vi "Escribir_Fichero_Registro.vi"(0 "refnum FILE":refnum<file>, 1 "ASIC QR CODE":string, 2 "HORA COMIENZO":timestamp, 3 "Coordenada X":string, 4 "Coordenada Y":string, 5 "OPERADOR":string, 6 "Resultado test":bool, 7 "error in (no error)":errorcluster) -> (20 "refnum out":refnum<file>, 27 "error out":errorcluster)   [LabVIEW 2019]
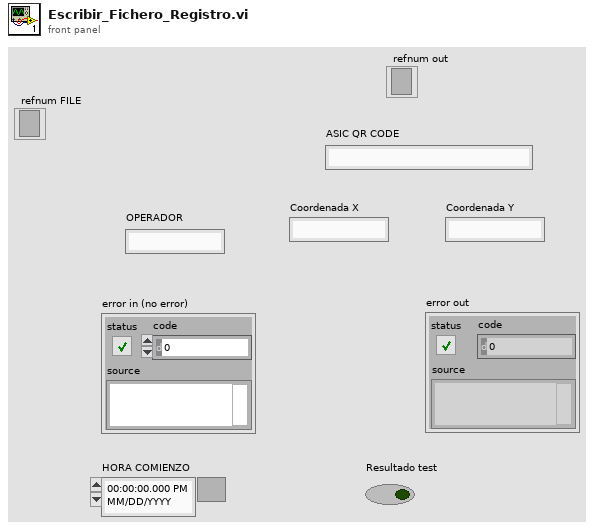
[diagram p1: front panel]
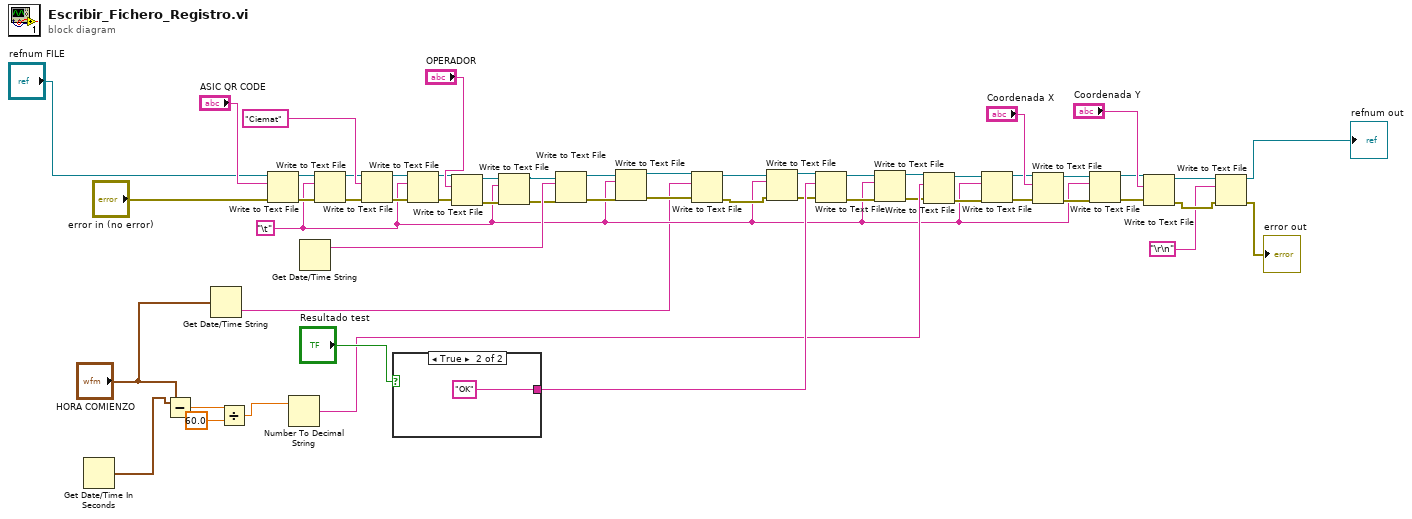
[diagram p0: block diagram]
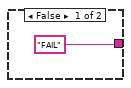
[diagram p2: hidden frame]
diagram:
  w5 = "\t"
  n1 = Get Date/Time In Seconds() -> (seconds since 1Jan1904=w48:timestamp)
  n2 = Subtract(x=w48, y="HORA COMIENZO") -> (x-y=w47:dbl)
  n3 = Get Date/Time String(seconds (now)="HORA COMIENZO") -> (time string=w1:string)  [unwired: 2 in, 1 out]
  n4 = Divide(x=w47, y=60.0) -> (x/y=w45:dbl)
  n5 = Write to Text File(file (use dialog)="refnum FILE", text="ASIC QR CODE", error in="error in (no error)") -> (refnum out=w35:refnum<file>, error out=w34:errorcluster)  [unwired: 1 in, 1 out]
  n6 = Number To Decimal String(number=w45) -> (decimal integer string=w44:string)  [unwired: 1 in]
  n7 = Get Date/Time String() -> (date string=w51:string)  [unwired: 3 in, 1 out]
  n8 = Write to Text File(file (use dialog)=w35, text=w5, error in=w34) -> (refnum out=w33:refnum<file>, error out=w32:errorcluster)  [unwired: 1 in, 1 out]
  n9 = Write to Text File(file (use dialog)=w33, text="Ciemat", error in=w32) -> (refnum out=w31:refnum<file>, error out=w30:errorcluster)  [unwired: 1 in, 1 out]
  n10 = case shown="True" "Resultado test" {
    tunnel: ["FAIL" "OK"] -> w49
    frame False {
    }
    frame True {
    }
  }
  n11 = Write to Text File(file (use dialog)=w31, text=w5, error in=w30) -> (refnum out=w29:refnum<file>, error out=w28:errorcluster)  [unwired: 1 in, 1 out]
  n12 = Write to Text File(file (use dialog)=w29, text="OPERADOR", error in=w28) -> (refnum out=w27:refnum<file>, error out=w26:errorcluster)  [unwired: 1 in, 1 out]
  n13 = Write to Text File(file (use dialog)=w27, text=w5, error in=w26) -> (refnum out=w25:refnum<file>, error out=w24:errorcluster)  [unwired: 1 in, 1 out]
  n14 = Write to Text File(file (use dialog)=w25, text=w51, error in=w24) -> (refnum out=w23:refnum<file>, error out=w22:errorcluster)  [unwired: 1 in, 1 out]
  n15 = Write to Text File(file (use dialog)=w23, text=w5, error in=w22) -> (refnum out=w21:refnum<file>, error out=w20:errorcluster)  [unwired: 1 in, 1 out]
  n16 = Write to Text File(file (use dialog)=w21, text=w1, error in=w20) -> (refnum out=w19:refnum<file>, error out=w18:errorcluster)  [unwired: 1 in, 1 out]
  n17 = Write to Text File(file (use dialog)=w19, text=w5, error in=w18) -> (refnum out=w17:refnum<file>, error out=w16:errorcluster)  [unwired: 1 in, 1 out]
  n18 = Write to Text File(file (use dialog)=w17, text=w49, error in=w16) -> (refnum out=w15:refnum<file>, error out=w14:errorcluster)  [unwired: 1 in, 1 out]
  n19 = Write to Text File(file (use dialog)=w15, text=w5, error in=w14) -> (refnum out=w12:refnum<file>, error out=w13:errorcluster)  [unwired: 1 in, 1 out]
  n20 = Write to Text File(file (use dialog)=w12, text=w44, error in=w13) -> (refnum out=w10:refnum<file>, error out=w11:errorcluster)  [unwired: 1 in, 1 out]
  n21 = Write to Text File(file (use dialog)=w10, text=w5, error in=w11) -> (refnum out=w9:refnum<file>, error out=w8:errorcluster)  [unwired: 1 in, 1 out]
  n22 = Write to Text File(file (use dialog)=w9, text="Coordenada X", error in=w8) -> (refnum out=w7:refnum<file>, error out=w6:errorcluster)  [unwired: 1 in, 1 out]
  n23 = Write to Text File(file (use dialog)=w7, text=w5, error in=w6) -> (refnum out=w4:refnum<file>, error out=w3:errorcluster)  [unwired: 1 in, 1 out]
  n24 = Write to Text File(file (use dialog)=w4, text="Coordenada Y", error in=w3) -> (refnum out=w41:refnum<file>, error out=w40:errorcluster)  [unwired: 1 in, 1 out]
  n25 = Write to Text File(file (use dialog)=w41, text="\r\n", error in=w40) -> (refnum out=→"refnum out":refnum<file>, error out=→"error out":errorcluster)  [unwired: 1 in, 1 out]
